vi "Send GOODBYE.vi"(8 "timeout ms (100)":i32=100, 9 "Termination Reason":T1, 10 "error in (no error)":errorcluster, 11 "WAMP Client in":refnum<class "WAMP Client.lvclass">) -> (2 "error out":errorcluster, 3 "WAMP Client out":refnum<class "WAMP Client.lvclass">)   [LabVIEW 2020, in "wamplv.lvlib" / "WAMP Client.lvclass"]
uses:
  WAMP Client.lvclass
  TypeDef/Termination Reason.ctl
  TypeDef/Termination Reason Enum.ctl
  WAMP Client.lvclass/WAMP Client.ctl
  Private/Comm Handlers/ICommHandler/ICommHandler.lvclass
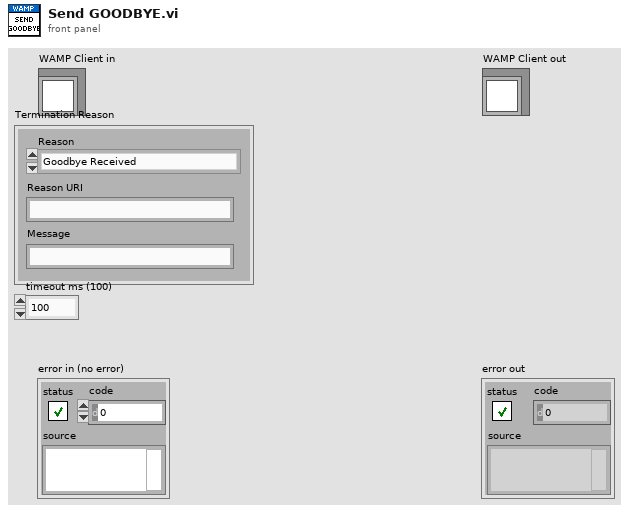
[diagram p1: front panel]
types:
  T1 = typedef "wamplv.lvlib/WAMP Client.lvclass/Termination Reason.ctl" = cluster{"Reason":T2, "Reason URI":string, "Message":string}
  T2 = typedef "wamplv.lvlib/WAMP Client.lvclass/Termination Reason Enum.ctl" = enum16{"Goodbye Received", "Abort Received", "Send Goodbye", "Send Abort", "Read Loop Failure", "Write Loop Failure", "Message Loop Failure"}
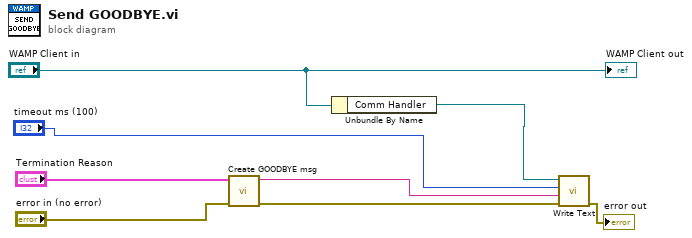
[diagram p0: block diagram]
diagram:
  n1 = call "Create GOODBYE msg.vi"("error in"="error in (no error)", "Termination Reason"="Termination Reason") -> ("error out"=w2:errorcluster, "String"=w4:string)  [unwired: 8 in]
  n2 = Unbundle By Name("WAMP Client in") -> ("Comm Handler"=w5:refnum<class "ICommHandler.lvclass">)
  n3 = call-dynamic "Write Text.vi"("error in (no error)"=w2, "String"=w4, "timeout ms (5000)"="timeout ms (100)", "ICommHandler in"=w5) -> ("error out"=→"error out":errorcluster)  [unwired: 6 in, 1 out]
  "WAMP Client out" <- "WAMP Client in"
